vi "GlobalReg.vi"() -> ()   [LabVIEW 2013, in "IRIO.lvlib"]
uses:
  IRIO.lvlib
  ctl/AcquisitionStateControl.ctl
panel:
  in  "Fix Value for AOs":bool
  out "DAQstate":T1
  out "Numeric 2":i16
  out "Numeric":i16
  out "AI2":i32
  out "AI1":i32
  out "AI0":i32
  out "DI2":bool
  out "DI1":bool
  out "DI0":bool
  in  "DO2":bool
  in  "DO1":bool
  in  "DO0":bool
  in  "AO2":i32
  in  "AOEnable2":bool
  out "auxDI6":bool
  in  "auxAI10":i32
  in  "auxAI9":i32
  in  "auxDO6":bool
  out "toDigPort":u8
  in  "SGUpdateRate0":u32=40
  in  "SGSignalType0":u8
  in  "SGPhase0":u32
  in  "SGFreq0":u32=100000
  in  "SGAmp0":u16
  in  "AO0":i32
  in  "SGSignalType1":u8
  in  "SGAmp1":u16
  in  "SGPhase1":u32
  in  "SGFreq1":u32=100000
  in  "SGUpdateRate1":u32=40
  in  "AO1":i32
  in  "AOEnable1":bool
  in  "AOEnable0":bool
  in  "SimulatedAO1":i32
  in  "SimulatedAO0":i32
  out "DMAsOverflow15":bool
  out "DMAsOverflow14":bool
  out "DMAsOverflow13":bool
  out "DMAsOverflow12":bool
  out "DMAsOverflow11":bool
  out "DMAsOverflow10":bool
  out "DMAsOverflow9":bool
  out "DMAsOverflow8":bool
  out "DMAsOverflow7":bool
  out "DMAsOverflow6":bool
  out "DMAsOverflow5":bool
  out "DMAsOverflow4":bool
  out "DMAsOverflow3":bool
  out "DMAsOverflow2":bool
  out "DMAsOverflow1":bool
  out "DMAsOverflow0":bool
  out "DMAsOverflow":u16
  in  "GroupEnable5":bool
  in  "SamplingRate5":u16=10000
  in  "GroupEnable4":bool
  in  "SamplingRate4":u16=10000
  in  "GroupEnable3":bool
  in  "SamplingRate3":u16=10000
  in  "GroupEnable2":bool
  in  "SamplingRate2":u16=10000
  in  "GroupEnable1":bool
  in  "SamplingRate1":u16=10000
  in  "GroupEnable0":bool
  in  "SamplingRate0":u16=10000
  in  "DebugMode":bool
  in  "DAQStartStop":bool
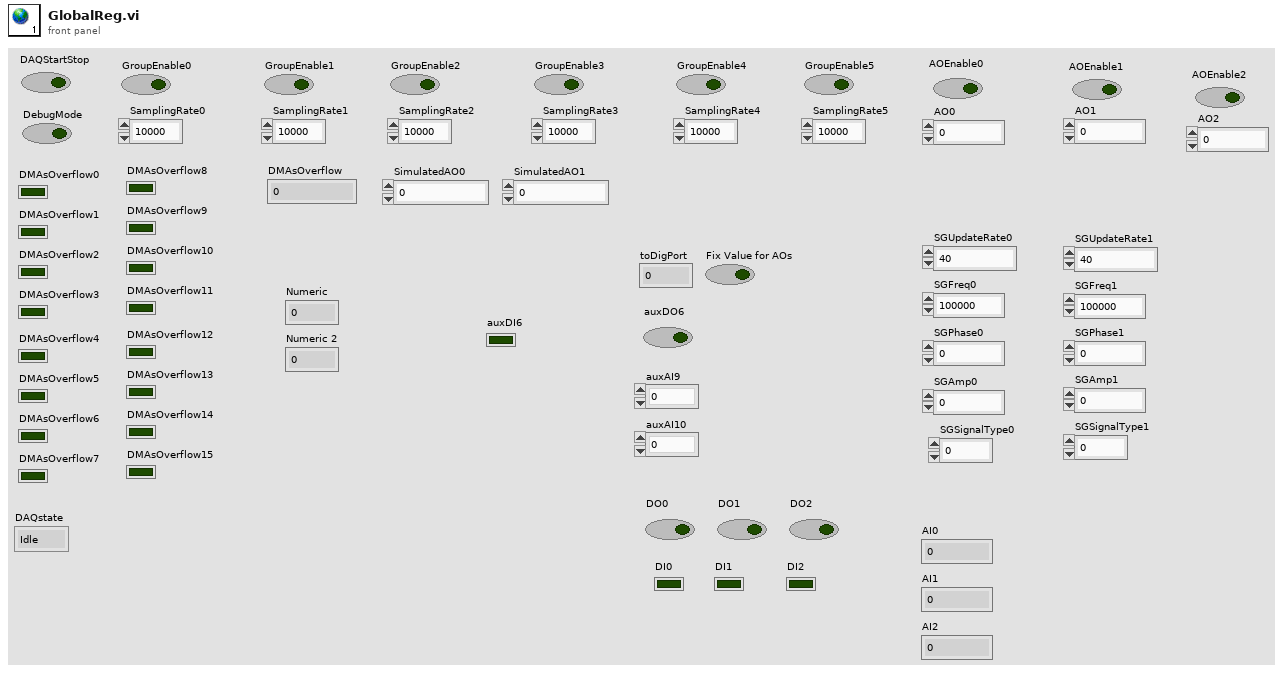
[diagram p1: front panel]
types:
  T1 = typedef "IRIO.lvlib/AcquisitionStateControl.ctl" = enum16{"Idle", "Acq"}
diagram:
